vi "Opgave 2 Tal match.vi"(9 "Maksimale værdi":i32=100, 10 "Mindste værdi":i32, 11 "Brugerbestemt tal":i32) -> (3 "Iterationer":i32)   [LabVIEW 2019]
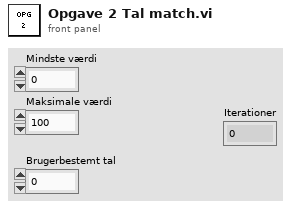
[diagram p1: front panel]
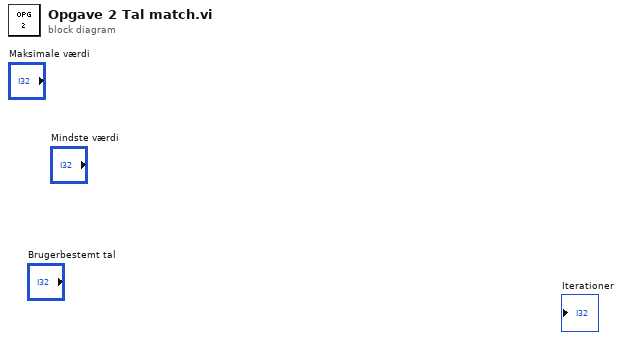
[diagram p0: block diagram]
diagram:
